vi "Configure Signaling TDD DL Flexible Slot Symbol.vi"(7 "Slot Symbol (0)":i32, 8 "error in (no error)":errorcluster, 9 "Pattern (1)":T1=1, 10 "Cell Name (\"Cell Name\")":string="Cell Name", 11 "VISA resource name":refnum<visa-resource-name>) -> (0 "error out":errorcluster, 3 "VISA resource name out":refnum<visa-resource-name>)   [LabVIEW 2020, in "Rohde&Schwarz CMWXP NR FR1 Measurement.lvlib"]
doc: "Defines the number of DL symbols in the flexible slot of the UL-DL pattern <p>.\n\nAttribute:\nRSCMWXPNRFR1M_ATTR_SIGNALING_TDD_DL_FLEXIBLE_SLOT_SYMBOL\n\nRemote-control command:\n[CONFigure:]SIGNaling:NRADio:CELL:TDD:PATTern<p>:DL:FSSYmbol"
uses:
  <instrlib>/Rohde&Schwarz CMWXP NR FR1 Measurement/Rohde&Schwarz CMWXP NR FR1 Measurement.lvlib
  <instrlib>/Rohde&Schwarz CMWXP NR FR1 Measurement/Private/_Pattern.ctl
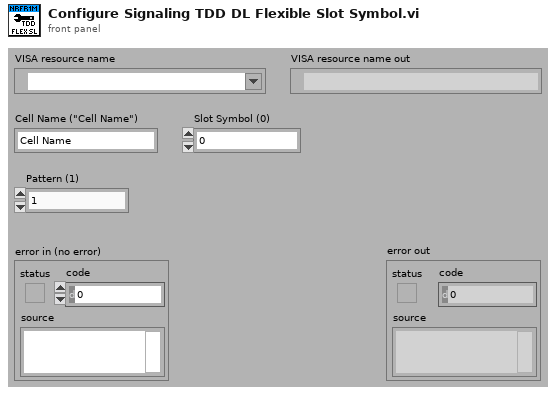
[diagram p1: front panel]
types:
  T1 = typedef "Rohde&Schwarz CMWXP NR FR1 Measurement.lvlib/_Pattern.ctl" = i32
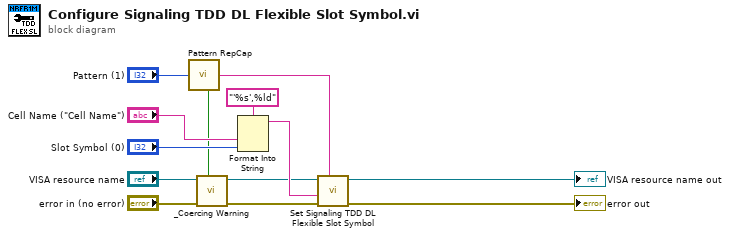
[diagram p0: block diagram]
diagram:
  n1 = call <instrlib>:"Pattern RepCap.vi"("Pattern In"="Pattern (1)") -> ("In Range?"=w1:bool, "RepCap Identifier Out"=w10:string)  [unwired: 1 in]
  n2 = call <instrlib>:"_Coercing Warning.vi"("In Range?"=w1, "error in (no error)"="error in (no error)", "VISA resource name"="VISA resource name") -> ("error out"=w3:errorcluster, "VISA resource name out"=w2:refnum<visa-resource-name>)  [unwired: 7 in]
  n3 = Format Into String(format string="'%s',%ld", "Cell Name (\"Cell Name\")", "Slot Symbol (0)") -> (resulting string=w6:string)  [unwired: 2 in, 1 out]
  n4 = call "Set Signaling TDD DL Flexible Slot Symbol"("Repeated Capabilities"=w10, "error in (no error)"=w3, "Signaling TDD DL Flexible Slot Symbol ()"=w6, "instrument handle"=w2) -> ("error out"=→"error out":errorcluster, "instrument handle out"=→"VISA resource name out":refnum<visa-resource-name>)  [unwired: 6 in]
